vi "data extraction from Arduino message.vi"(0 "data (can be any type)":string="#123#45#34#67&1&0", 11 "error IO":errorcluster) -> (3 "size analog array":i32, 4 "DIn 0":bool, 6 "Analog channel reading":u32[](array[numeric]), 8 "DIn 1":bool, 10 "digital input state":u32[](array[numeric]), 14 "size digital array":i32, 15 "error out":errorcluster)   [LabVIEW 2018]
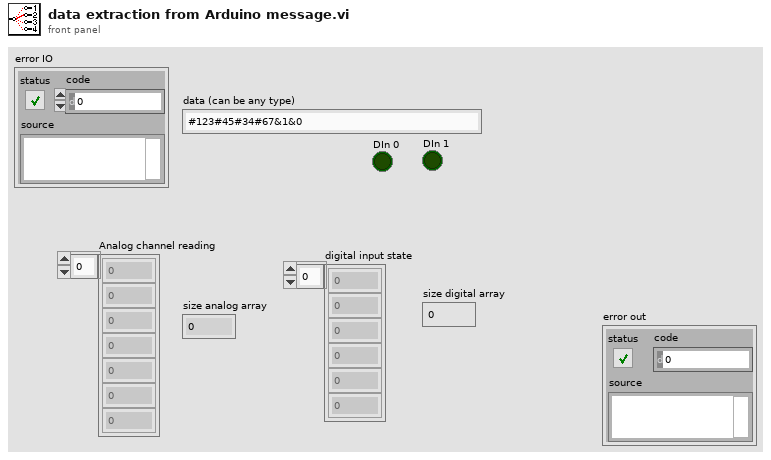
[diagram p1: front panel]
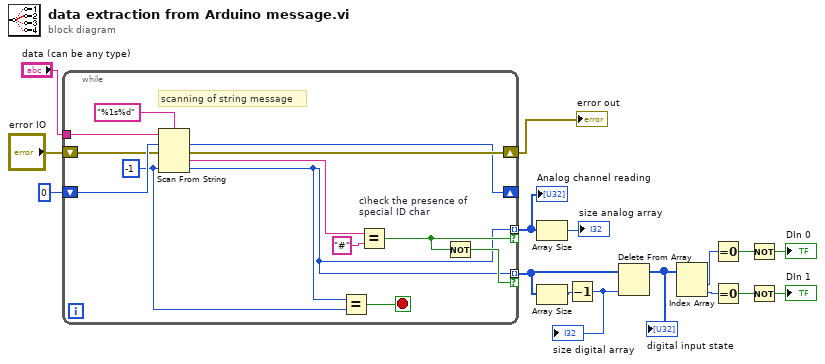
[diagram p0: block diagram]
diagram:
  n1 = while {
    tunnel: "data (can be any type)" -> [w29]
    shift-right: [w20] -> _
    shift-left: u32 0 -> [w27]
    shift-right: [w26] -> w1
    shift-left: "error IO" -> [w25]
    tunnel: [w17] -> w2 mode=indexing if=w19
    tunnel: [w17] -> w8 mode=indexing if=w18
    stop <- w23 stop-if-true
    w24 = -1 ("default value 2")
    # "scanning of string message"
    n2 = Scan From String(format string="%1s%d", input string=w29, initial scan location=w27, error in=w25, default 2=w24) -> (offset past scan=w20:u32, error out=w26:errorcluster, output 1=w22:string, output 2=w17:i32)  [unwired: 1 in, 1 out]
    n3 = Equal?(x=w17, y=w24) -> (x = y?=w23:bool)
    n4 = Equal? "cìheck the presence of \nspecial ID char"(x=w22, y="#") -> (x = y?=w19:bool)
    n5 = Not(x=w19) -> (.not. x?=w18:bool)
  }
  "Analog channel reading" <- w2
  "error out" <- w1
  n6 = Array Size(array=w2) -> (size(s)=→"size analog array":i32)
  n7 = Array Size(array=w8) -> (size(s)=w6:i32)
  n8 = Decrement(x=w6) -> (x-1=w5:i32)
  "size digital array" <- w5
  n9 = Delete From Array(array=w8, index=w5) -> (array with subset deleted=w7:i32[])  [unwired: 1 in, 1 out]
  "digital input state" <- w7
  n10 = Index Array(array=w7) -> (element #1=w13:i32, element #2=w4:i32)  [unwired: 2 in]
  n11 = Equal To 0?(x=w13) -> (x = 0?=w12:bool)
  n12 = Equal To 0?(x=w4) -> (x = 0?=w11:bool)
  n13 = Not(x=w12) -> (.not. x?=→"DIn 0":bool)
  n14 = Not(x=w11) -> (.not. x?=→"DIn 1":bool)
